vi "Find Relative Goal Location.vi"(0 "Current Position":T1 {"Time"."GPS Time of Week" format="%.3f"; "Velocity, Correction & SET"."Extended Navigation Mode" items=["Non Differential"=0, "Code (RTCM Type 1 & 9)"=1, "Code, Single Frequency (WAAS)"=2, "Code, Dual Frequency (WAAS)"=3, "Code, Single Frequency (WCT)"=4, "Code/RCP, Dual Frequency (WCT)"=5, "Code, Single Frequency (RTG)"=6, "Code (RTCM Type 1 & 9) Dual Frequency"=10, "Code/RCP, Dual Frequency (RTG)"=11, "Code, Single Frequency (NCT-RTK)"=12, "Code, Single Frequency (RTCM 18 & 19)"=13, "Code, Single Frequency (RTCM 21 & 22)"=14, "Code, Single Frequency (CMR)"=15, "Code, Dual Frequency (NCT-RTK)"=16, "Code, Dual Frequency (RTCM 18 & 19)"=17, "Code, Dual Frequency (RTCM 20 & 21)"=18, "Code, Dual Frequency (CMR)"=19, "RTK (NCT-RTK)"=20, "RTK (RTCM 18 & 19)"=21, "RTK (RTCM 20 & 21)"=22, "RTK (CMR)"=23, "Code, Single Frequency with SET (RTG)"=24, "Code/RCP, Dual Frequency with SET (RTG)"=25, "RTK Extend"=26]}, 1 "Goal Position":T1 {"Time"."GPS Time of Week" format="%.3f"; "Velocity, Correction & SET"."Extended Navigation Mode" items=["Non Differential"=0, "Code (RTCM Type 1 & 9)"=1, "Code, Single Frequency (WAAS)"=2, "Code, Dual Frequency (WAAS)"=3, "Code, Single Frequency (WCT)"=4, "Code/RCP, Dual Frequency (WCT)"=5, "Code, Single Frequency (RTG)"=6, "Code (RTCM Type 1 & 9) Dual Frequency"=10, "Code/RCP, Dual Frequency (RTG)"=11, "Code, Single Frequency (NCT-RTK)"=12, "Code, Single Frequency (RTCM 18 & 19)"=13, "Code, Single Frequency (RTCM 21 & 22)"=14, "Code, Single Frequency (CMR)"=15, "Code, Dual Frequency (NCT-RTK)"=16, "Code, Dual Frequency (RTCM 18 & 19)"=17, "Code, Dual Frequency (RTCM 20 & 21)"=18, "Code, Dual Frequency (CMR)"=19, "RTK (NCT-RTK)"=20, "RTK (RTCM 18 & 19)"=21, "RTK (RTCM 20 & 21)"=22, "RTK (CMR)"=23, "Code, Single Frequency with SET (RTG)"=24, "Code/RCP, Dual Frequency with SET (RTG)"=25, "RTK Extend"=26]}) -> (2 "Target Heading (deg)":dbl, 3 "Target Heading (rad)":dbl, 4 "Target Distance":dbl)   [LabVIEW 2012]
uses:
  <vilib>/imath/engines/lvmath2/RunTimeEngine/NodeEndStatement/NIMS_NodeEndStatement_Output.vi
  <instcachedir>/0/NIMS_NodeEndStatement_Output_53EC0D466D134D7ABD903AC30B43404B.lvgen/NIMS_NodeEndStatement_Output_53EC0D466D134D7ABD903AC30B43404B_001.vi
  <vilib>/imath/engines/lvmath2/RunTimeEngine/BuiltInFunctions/atan2/NIMS_atan2.vi
  <instcachedir>/0/NIMS_atan2_A91AA4A7D42247EDBE8F76DB99AF04A4.lvgen/NIMS_atan2_A91AA4A7D42247EDBE8F76DB99AF04A4_000.vi
  <instcachedir>/0/NIMS_atan2_A91AA4A7D42247EDBE8F76DB99AF04A4.lvgen/NIMS_atan2_A91AA4A7D42247EDBE8F76DB99AF04A4_001.vi
  <vilib>/imath/engines/lvmath2/RunTimeEngine/ErrorHandling/NIMS_Finalize Error.vi
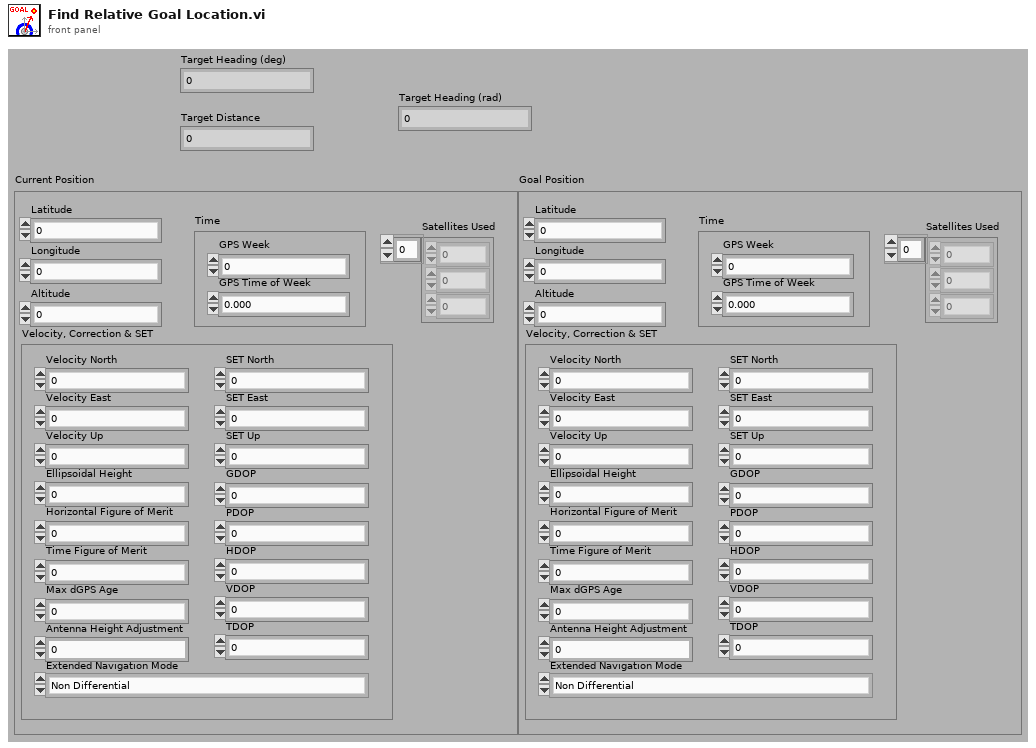
[diagram p1: front panel]
types:
  T1 = cluster{"Latitude":dbl, "Longitude":dbl, "Altitude":dbl, "Velocity, Correction & SET":cluster{"Velocity North":dbl, "Velocity East":dbl, "Velocity Up":dbl, "Ellipsoidal Height":dbl, "GDOP":sgl, "PDOP":sgl, "HDOP":sgl, "VDOP":sgl, "TDOP":sgl, "Horizontal Figure of Merit":u8, "Time Figure of Merit":u8, "Max dGPS Age":sgl, "Extended Navigation Mode":u8, "Antenna Height Adjustment ":dbl, "SET North":i32, "SET East":i32, "SET Up":i32}, "Time":cluster{"GPS Week":u16, "GPS Time of Week":sgl}, "Satellites Used":i32[]}
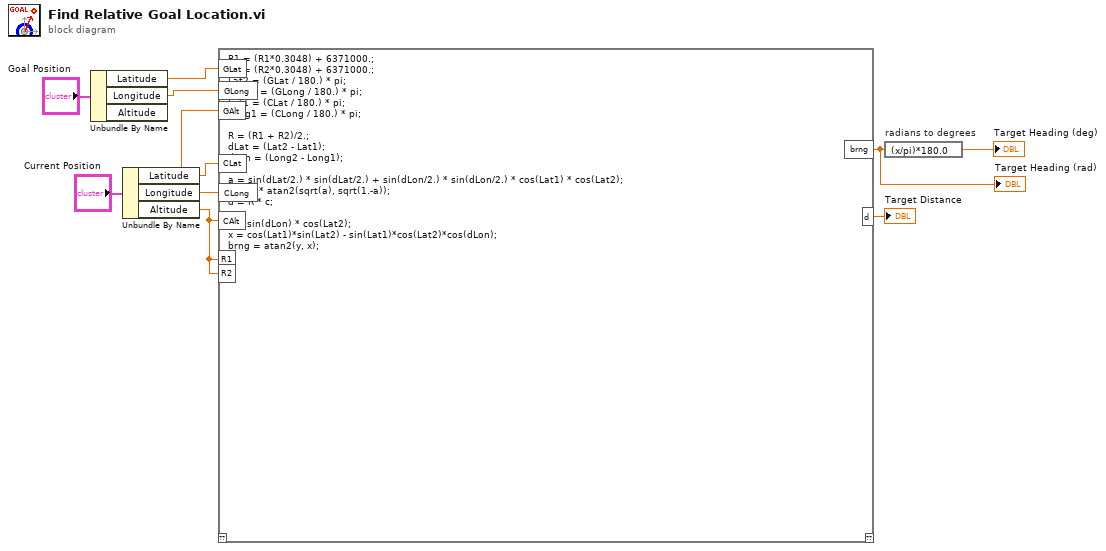
[diagram p0: block diagram]
diagram:
  n1 = Unbundle By Name("Goal Position") -> ("Latitude"=w8:dbl, "Longitude"=w7:dbl)  [unwired: 1 out]
  n2 = Unbundle By Name("Current Position") -> ("Latitude"=w6:dbl, "Longitude"=w5:dbl, "Altitude"=w1:dbl)
  n3 = mathscript code="R1 = (R1*0.3048) +\t6371000.;\nR2 = (R2*0.3048) +\t6371000.;\nLat2 = (GLat / 180.) * pi;\nLong2 = (GLong / 180.) * pi;\nLat1 = (CLat / 180.) * pi;\nLong1 = (CLong / 180.) * pi;\n\nR = (R1 + R2)/2.; \ndLat = (Lat2 - Lat1);\ndLon = (Long2 - Long1);\n\na = sin(dLat/2.) * sin(dLat/2.) + sin(dLon/2.) * sin(dLon/2.) * cos(Lat1) * cos(Lat2); \nc = 2. * atan2(sqrt(a), sqrt(1.-a)); \nd = R * c;\n\ny = sin(dLon) * cos(Lat2);\nx = cos(Lat1)*sin(Lat2) - sin(Lat1)*cos(Lat2)*cos(dLon);\nbrng = atan2(y, x);"("GLong"=w7, "GLat"=w8, "GAlt"=w1, "CLat"=w6, "CLong"=w5, "CAlt"=w1, "R1"=w1, "R2"=w1) -> ("brng"=w2:dbl, "d"=→"Target Distance":dbl)  [unwired: 1 in, 1 out]
  "Target Heading (rad)" <- w2
  n4 = expression code="(x/pi)*180.0" "radians to degrees"(w2) -> (→"Target Heading (deg)":dbl)
